vi "Actor Core.vi"(8 "error in":errorcluster, 11 "KIT-QVA in":refnum<class "KIT-QVA.lvclass">) -> (0 "error out":errorcluster, 3 "Actor out":refnum<class "Actor.lvclass">)   [LabVIEW 2015, in "KIT-QVA.lvlib" / "KIT-QVA.lvclass"]
doc: "(<B>Filename</B>: Actor Framework.lvlib:Actor.lvclass:Actor Core.vi)\n\nReceives messages to the actor, reacts to them, and initiates any error handling that may shut the actor down.\n\nDescendant classes may override this VI to append parallel tasks for the actor to complete while it handles messages. Overrides use the Call Parent Method node."
uses:
  KIT-QVA.lvclass
  <vilib>/ActorFramework/Actor/Actor.lvclass
  CSPP_Core/Actors/CS++BaseActor/CS++BaseActor.lvclass/CS++BaseActor.ctl
  KIT-QVA.lvclass/KIT-QVA.ctl
  <vilib>/ActorFramework/Actor/Actor.lvclass/Actor.ctl
  <vilib>/ActorFramework/Message Enqueuer/Message Enqueuer.lvclass/Message Enqueuer.ctl
  KIT-QVA Messages/Control Mode Msg/Control Mode Msg.lvclass/Control Mode Msg.ctl
  KIT-QVA Messages/Quench Msg/Quench Msg.lvclass/Quench Msg.ctl
  KIT-QVA Messages/Acknowledge Fault Msg/Acknowledge Fault Msg.lvclass/Acknowledge Fault Msg.ctl
  <vilib>/ActorFramework/Message Enqueuer/Enqueue.vi
  <vilib>/ActorFramework/Message Enqueuer/Init from Existing Queue.vi
  <vilib>/ActorFramework/Message Priority Queue/Priority Enqueue.vi
  KIT-QVA Messages/Acknowledge Fault Msg/Acknowledge Fault Msg.lvclass
  KIT-QVA Messages/Quench Msg/Quench Msg.lvclass
  KIT-QVA Messages/Control Mode Msg/Control Mode Msg.lvclass
  <vilib>/ActorFramework/Stop Msg/Stop Msg.lvclass
  <vilib>/ActorFramework/Message Enqueuer/Message Enqueuer.lvclass
  CSPP_Core/Actors/CS++DeviceActor/CS++DeviceActor.lvclass
  CSPP_Core/Actors/CS++BaseActor/CS++BaseActor.lvclass
  CSPP_Core/Libraries/Utilities/CS++Utilities.lvlib
panel:
  out "KIT-QV-Status":T1={"Last Update"=timestamp(0 s since 1904-01-01), "Rack Status"={"System Test"=FALSE, "Test Mode"=FALSE, "Fault"=FALSE, "Quench"=FALSE, "U/T Fault"=FALSE, "Bus Error"=FALSE, "System Fault"=FALSE, "Control Mode"=FALSE}, "Update if in control mode"={"Last Update"=timestamp(0 s since 1904-01-01), "Temperature"=273.15, "Detectors"=[]}} {"Update if in control mode"."Detectors"."Voltage" format="%.4f"; "Update if in control mode"."Last Update" format="%<%H:%M:%S\n%d/%m/%Y>T"; "Last Update" format="%<%H:%M:%S\n%d/%m/%Y>T"}
  in  "Stop Button":bool
  in  "Quench":bool
  in  "FQuit":bool
  in  "Stop":bool
  in  "Start":bool
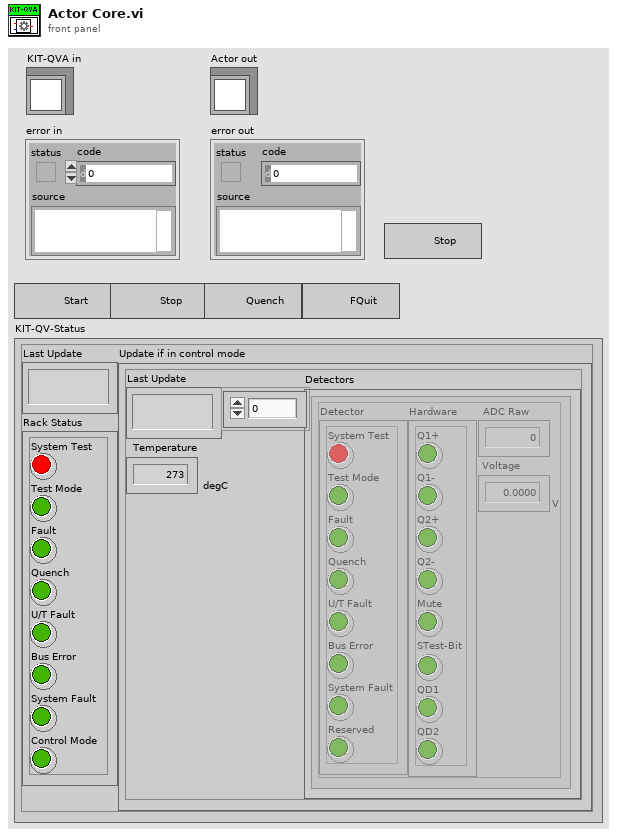
[diagram p1: front panel]
types:
  T1 = cluster{"Last Update":timestamp, "Rack Status":cluster{"System Test":bool, "Test Mode":bool, "Fault":bool, "Quench":bool, "U/T Fault":bool, "Bus Error":bool, "System Fault":bool, "Control Mode":bool}, "Update if in control mode":cluster{"Last Update":timestamp, "Temperature":dbl[unit], "Detectors":cluster{"Detector":cluster{"System Test":bool, "Test Mode":bool, "Fault":bool, "Quench":bool, "U/T Fault":bool, "Bus Error":bool, "System Fault":bool, "Reserved":bool}, "Hardware":cluster{"Q1+":bool, "Q1-":bool, "Q2+":bool, "Q2-":bool, "Mute":bool, "STest-Bit":bool, "QD1":bool, "QD2":bool}, "ADC Raw":i16, "Voltage":dbl[unit]}[]}}
  T2 = cluster{"Last Update":timestamp, "Rack Status":cluster{"System Test":bool, "Test Mode":bool, "Fault":bool, "Quench":bool, "U/T Fault":bool, "Bus Error":bool, "System Fault":bool, "Control Mode":bool}, "Update if in control mode":cluster{"Last Update":timestamp, "Temperature":dbl[unit], "Detectors":cluster{"Detector":cluster{"System Test":bool, "Test Mode":bool, "Fault":bool, "Quench":bool, "U/T Fault":bool, "Bus Error":bool, "System Fault":bool, "Reserved":bool}, "Hardware":cluster{"Q1+":bool, "Q1-":bool, "Q2+":bool, "Q2-":bool, "Mute":bool, "STest-Bit":bool, "QD1":bool, "QD2":bool}, "ADC Raw":i16, "Volatage":dbl[unit]}[]}}
  T3 = enum32{"Invalid", "Standard", "Closed", "Hidden", "Minimized", "Maximized"}
  T4 = cluster{"System Test":bool, "Test Mode":bool, "Fault":bool, "Quench":bool, "U/T Fault":bool, "Bus Error":bool, "System Fault":bool, "Control Mode":bool}
  T5 = cluster{"Last Update":timestamp, "Temperature":dbl[unit], "Detectors":cluster{"Detector":cluster{"System Test":bool, "Test Mode":bool, "Fault":bool, "Quench":bool, "U/T Fault":bool, "Bus Error":bool, "System Fault":bool, "Reserved":bool}, "Hardware":cluster{"Q1+":bool, "Q1-":bool, "Q2+":bool, "Q2-":bool, "Mute":bool, "STest-Bit":bool, "QD1":bool, "QD2":bool}, "ADC Raw":i16, "Volatage":dbl[unit]}[]}
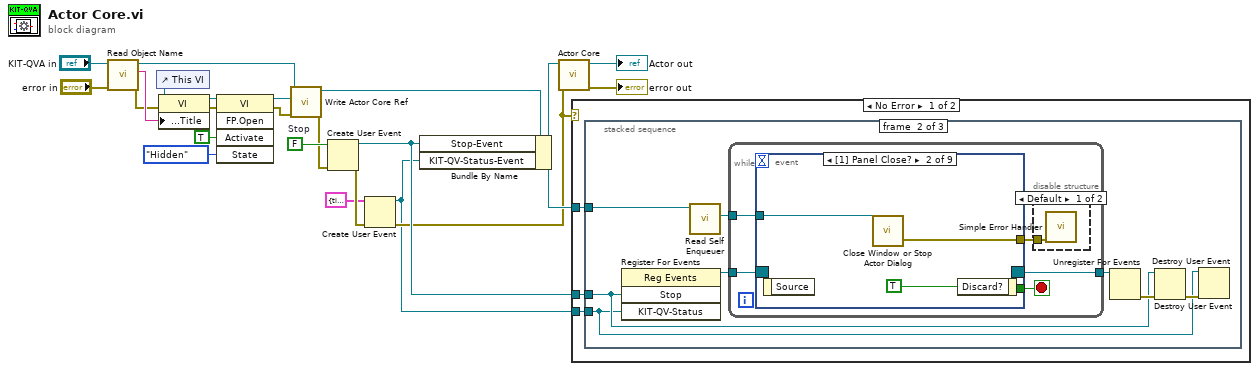
[diagram p0: block diagram]
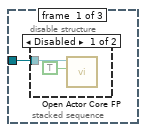
[diagram p2: hidden frame]
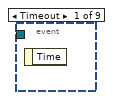
[diagram p5: hidden frame]
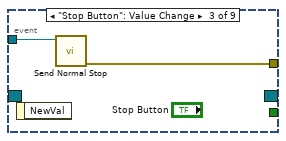
[diagram p6: hidden frame]
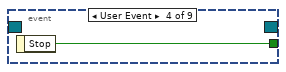
[diagram p7: hidden frame]
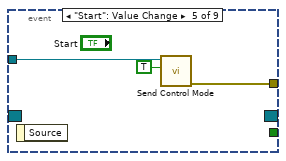
[diagram p8: hidden frame]
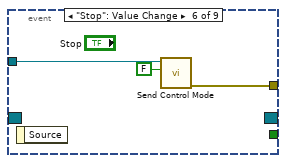
[diagram p9: hidden frame]
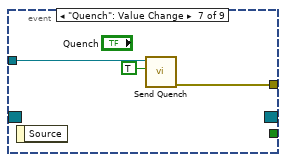
[diagram p10: hidden frame]
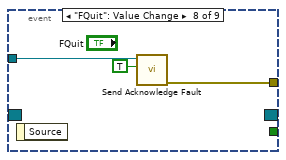
[diagram p11: hidden frame]
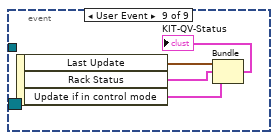
[diagram p12: hidden frame]
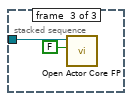
[diagram p13: hidden frame]
diagram:
  w9 = FALSE  # Stop
  n1 = call "Read Object Name.vi"("error in (no error)"="error in", "CS++BaseActor in"="KIT-QVA in") -> ("error out"=w10:errorcluster, "Object Name"=w11:string, "CS++BaseActor out"=w12:refnum<class "KIT-QVA.lvclass">)  [unwired: 7 in]
  n2 = control-ref of="This VI"() -> (w15:refnum<vi>)
  n3 = property class="VI"(reference=w15, error in=w10, "Front Panel.Title"=w11) -> (reference out=w14:refnum<vi>, error out=w13:errorcluster)
  n4 = invoke class="VI" method="FP.Open"(reference=w14, error in=w13, "Activate"=TRUE ("Activate?"), "State"=T3."Hidden") -> (reference out=w17:refnum<vi>, error out=w16:errorcluster)  [unwired: 1 in, 3 out]
  n5 = call "Write Actor Core Ref.vi"("error in (no error)"=w16, "Actor Core Ref"=w17, "CS++BaseActor in"=w12) -> ("error out"=w7:errorcluster, "CS++BaseActor out"=w8:refnum<class "KIT-QVA.lvclass">)  [unwired: 7 in]
  n6 = Create User Event(user event datatype=w9, error in=w7) -> (user event=w5:refnum<user-event>, error out=w4:errorcluster)
  n7 = Create User Event(user event datatype=T2 {"Last Update"=timestamp(0 s since 1904-01-01), "Rack Status"={"System Test"=FALSE, "Test Mode"=FALSE, "Fault"=FALSE, "Quench"=FALSE, "U/T Fault"=FALSE, "Bus Error"=FALSE, "System Fault"=FALSE, "Control Mode"=FALSE}, "Update if in control mode"={"Last Update"=timestamp(0 s since 1904-01-01), "Temperature"=273.15, "Detectors"=[]}} ("KIT-QV-Status"), error in=w4) -> (user event=w2:refnum<user-event>, error out=w3:errorcluster)
  n8 = Bundle By Name(cluster=w8, "Stop-Event"=w5, "KIT-QV-Status-Event"=w2) -> (w6:refnum<class "KIT-QVA.lvclass">)
  n9 = call-parent "Actor Core.vi"("error in"=w3, "CS++BaseActor in"=w6) -> ("error out"=→"error out":errorcluster, "Actor out"=→"Actor out":refnum<class "Actor.lvclass">)  [unwired: 8 in]
  n10 = case shown="No Error" w3 {
    tunnel: w6 -> [w26 _]
    tunnel: w5 -> [w25 _]
    tunnel: w2 -> [w24 _]
    frame No Error {
      n11 = stacked-sequence {
        tunnel: w26 -> [w27 w34 w67]
        tunnel: w25 -> [_ w31 _]
        tunnel: w24 -> [_ w30 _]
        frame #0 {
          n12 = disable-structure shown="Disabled" {
            disable-tunnel: w27 -> [w29 _]
            frame Disabled {
              n13 = call "Open Actor Core FP.vi"("Open FP (F)"=TRUE, "CS++BaseActor in"=w29) -> ()  [unwired: 8 in, 2 out]
            }
            frame Enabled {
            }
          }
        }
        frame #1 {
          n14 = register-events(w31, w30) -> (reference out=w35:refnum<event-registration>)  [unwired: 2 in, 1 out]
          n15 = call <vilib>:"Read Self Enqueuer.vi"("Actor"=w34) -> ("Self Enqueuer"=w36:refnum<class "Message Enqueuer.lvclass">)  [unwired: 10 in]
          n16 = while {
            tunnel: w35 -> [w42]
            tunnel: [w40] -> w37
            tunnel: w36 -> [w38]
            stop <- w41 stop-if-true
            n17 = event shown="[1] Panel Close?" {
              selector: w42 -> [_ _ _ _ _ _ _ _ _]
              dyn-events: [_ _ _ _ _ _ _ _ _] -> w40
              timeout: _ -> [_ _ _ _ _ _ _ _ _]
              tunnel: [_ _ _ w49 _ _ _ _ _] -> w41
              tunnel: [_ w44 w48 _ w50 w53 w57 w60 _] -> w39
              tunnel: w38 -> [_ w45 w47 _ w52 w55 w58 w61 _]
              event Timeout {
                n18 = event-data() -> ()  [unwired: 1 in, 1 out]
              }
              event Panel Close? {
                n19 = event-data() -> ()  [unwired: 1 in, 1 out]
                n20 = call "Close Window or Stop Actor Dialog.vi"("Self Enqueuer"=w45) -> ("Error Out"=w44:errorcluster)  [unwired: 2 in]
                n21 = event-data("Discard?"=TRUE) -> ()  [unwired: 1 in, 1 out]
              }
              event "Stop Button": Value Change {
                n22 = event-data() -> ()  [unwired: 1 in, 1 out]
                n23 = call <vilib>:"Send Normal Stop.vi"("Message Enqueuer"=w47) -> ("error out"=w48:errorcluster)  [unwired: 10 in]
              }
              event User Event {
                n24 = event-data() -> ("Stop"=w49:bool)  [unwired: 1 in]
              }
              event "Start": Value Change {
                n25 = event-data() -> ()  [unwired: 1 in, 1 out]
                n26 = call "Send Control Mode.vi"("Control Mode"=TRUE, "Message Enqueuer"=w52) -> ("error out"=w50:errorcluster)  [unwired: 8 in, 1 out]
              }
              event "Stop": Value Change {
                n27 = event-data() -> ()  [unwired: 1 in, 1 out]
                n28 = call "Send Control Mode.vi"("Control Mode"=FALSE, "Message Enqueuer"=w55) -> ("error out"=w53:errorcluster)  [unwired: 8 in, 1 out]
              }
              event "Quench": Value Change {
                n29 = event-data() -> ()  [unwired: 1 in, 1 out]
                n30 = call "Send Quench.vi"("Quench"=TRUE, "Message Enqueuer"=w58) -> ("error out"=w57:errorcluster)  [unwired: 8 in, 1 out]
              }
              event "FQuit": Value Change {
                n31 = event-data() -> ()  [unwired: 1 in, 1 out]
                n32 = call "Send Acknowledge Fault.vi"("Acknowledge Fault"=TRUE, "Message Enqueuer"=w61) -> ("error out"=w60:errorcluster)  [unwired: 8 in, 1 out]
              }
              event User Event {
                n33 = event-data() -> ("Last Update"=w65:timestamp, "Rack Status"=w64:T4, "Update if in control mode"=w63:T5)  [unwired: 1 in]
                n34 = Bundle("Last Update"=w65, "Rack Status"=w64, "Update if in control mode"=w63) -> (→"KIT-QV-Status":T2)  [unwired: 1 in]
              }
            }
            n35 = disable-structure shown="Default" {
              disable-tunnel: w39 -> [w43 _]
              frame condition #0 (active) {
                n36 = call <vilib>:"Simple Error Handler.vi"("error in (no error)"=w43) -> ()  [unwired: 4 in, 5 out]
              }
              frame condition #1 {
              }
            }
          }
          n37 = Unregister For Events(event registration refnum=w37) -> (error out=w33:errorcluster)  [unwired: 1 in]
          n38 = Destroy User Event(user event=w31, error in=w33) -> (error out=w32:errorcluster)
          n39 = Destroy User Event(user event=w30, error in=w32) -> ()  [unwired: 1 out]
        }
        frame #2 {
          n40 = call "Open Actor Core FP.vi"("Open FP (F)"=FALSE, "CS++BaseActor in"=w67) -> ()  [unwired: 8 in, 2 out]
        }
      }
    }
    frame Error {
    }
  }
